vi "Drive Loop Gyro Angle.vi"(10 "Yaw Wind":dbl, 11 "Drive Loop Cluster":T1) -> ()   [LabVIEW 2015]
uses:
  <userlib>/836-Library/Drive/Drive Code/Drive Code Support/Drive Code Bundle.ctl
  <userlib>/836-Library/Drive/Drive Code/Drive Code Support/Sensor Cluster.ctl
  <userlib>/836-Library/Drive/Drive Code/Drive Code Support/Camera Cluster.ctl
  <userlib>/836-Library/Drive/Drive Code/Drive Code Support/Drive Code Notifier.ctl
  <userlib>/836-Library/Drive/Drive Code/Drive Code Support/Drive Code Command.ctl
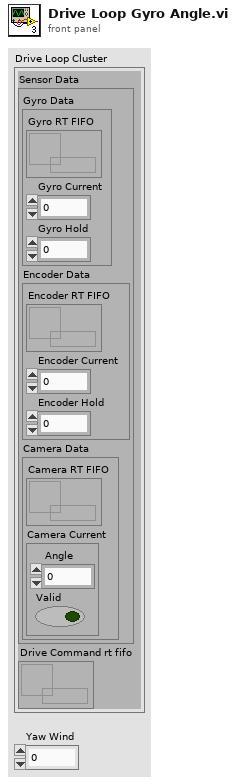
[diagram p1: front panel]
types:
  T1 = typedef "Drive Code Bundle.ctl" = cluster{"Sensor Data":T2, "Drive Command rt fifo":refnum<k33>}
  T2 = typedef "Sensor Cluster.ctl" = cluster{"Gyro Data":cluster{"Gyro RT FIFO":refnum<k33>, "Gyro Current":dbl, "Gyro Hold":dbl}, "Encoder Data":cluster{"Encoder RT FIFO":refnum<k33>, "Encoder Current":dbl, "Encoder Hold":dbl}, "Camera Data":cluster{"Camera RT FIFO":refnum<k33>, "Camera Current":T3}}
  T3 = typedef "Camera Cluster.ctl" = cluster{" Angle":dbl, "Valid":bool}
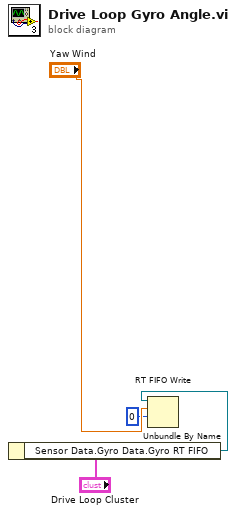
[diagram p0: block diagram]
diagram:
  n1 = Unbundle By Name("Drive Loop Cluster") -> ("Sensor Data.Gyro Data.Gyro RT FIFO"=w4:refnum<k33>)
  n2 = RT FIFO Write(0:w4, 1:"Yaw Wind", 2:0 ("timeout in ms (0)")) -> ()  [unwired: 2 in, 4 out]
